vi "Bronkhorst ProPar.vi"() -> ()   [LabVIEW 2015]
doc: "Example VI that demonstrates library features."
uses:
  PL Bronkhorst ProPar.lvclass
panel:
  out "fluid name":string
  out "device model":string
  in  "wink":bool
  in  "reset":bool
  out "temperature, °C":sgl
  out "sensor type":u8(ring) items=["pressure (controller)"=0, "liquid volume (controller)"=1, "liquid/gas mass (controller)"=2, "gas volume (controller)"=3, "other sensor type (controller)"=4, "pressure (sensor)"=128, "liquid volume (sensor)"=129, "liquid/gas mass (sensor)"=130, "gas volume (sensor)"=131, "other sensor type (sensor)"=132]
  out "device type":string
  in  "control mode":u8(ring) items=["setpoint = BUS setpoint", "setpoint = analog input", "setpoint = master output(FLOW-BUS) * slave factor(FLOW-BUS)", "close valve", "controller idle", "testmode enable", "tuningmode enable", "setpoint = 100%", "purge valve", "calibration mode enable", "setpoint = master output(analog in) * slave factor(FLOW-BUS)", "setpoint = keyboard OR FLOW-BUS setpoint", "setpoint = 0%", "setpoint = master output(FLOW-BUS) * slave factor(analog in)", "(FPP) range select mode", "(FPP) manual start sensor select, automatic end sensor", "(FPP) automatic start sensor select, manual end sensor", "(FPP) automatic start and end sensor", "setpoint = RS232 setpoint", "RS232 broadcast mode", "valve stearing", "analog valve stearing", "valve safe state"]
  out "counter unit":string
  in  "counter value":sgl
  out "capacity":sgl
  in  "setpoint":sgl
  out "capacity unit":string
  out "measured value":sgl
  out "firmware version":string
  in  "user tag":string
  out "id string":string
  in  "node":u8
  out "ProPar":refnum<class "PL Bronkhorst ProPar.lvclass">
  in  "baud rate":u32=38400
  in  "port":refnum<visa-resource-name>
  out "error":errorcluster
  in  "stop":bool
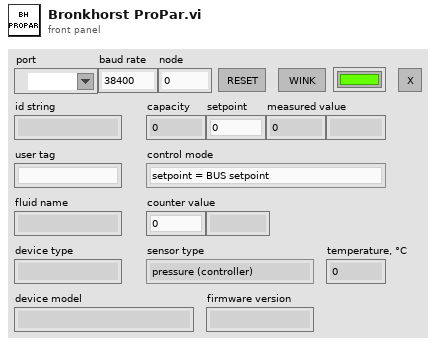
[diagram p1: front panel]
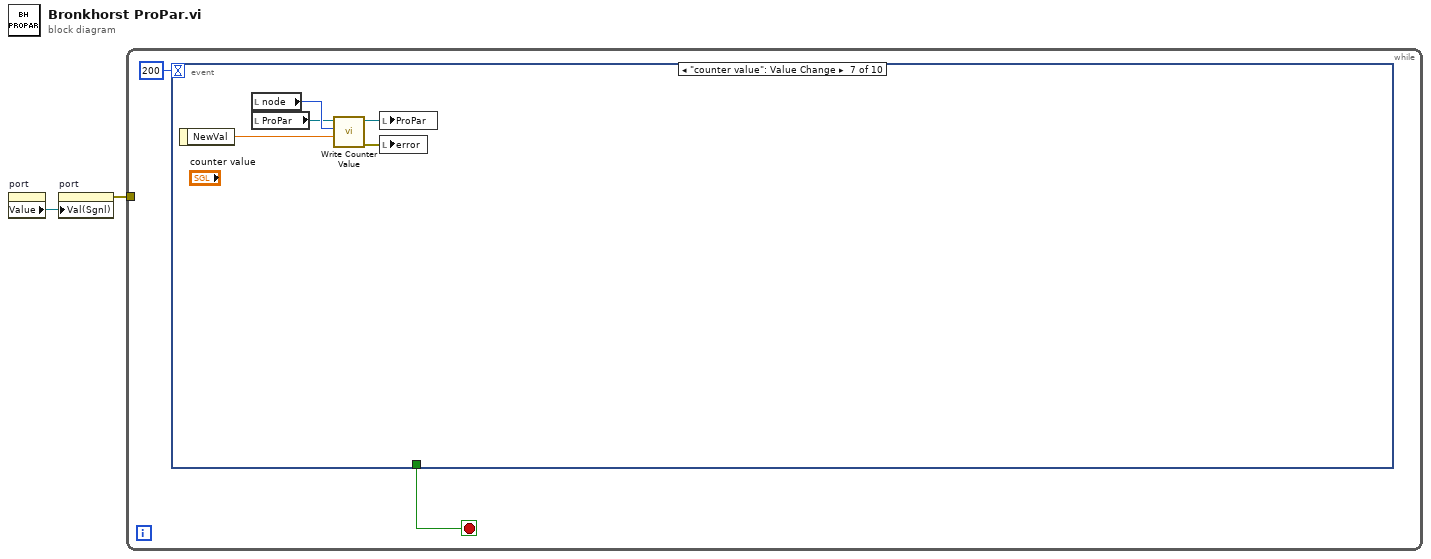
[diagram p0: block diagram]
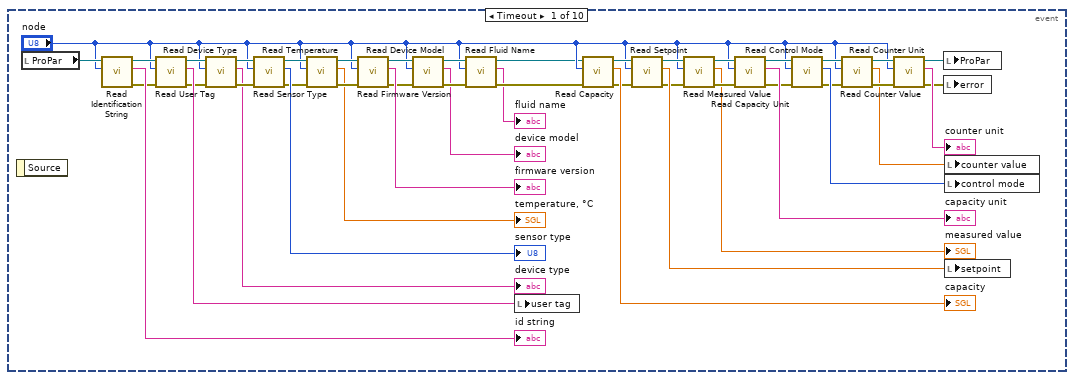
[diagram p2: hidden frame]
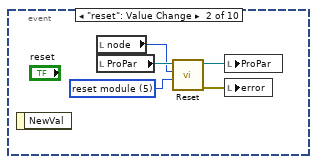
[diagram p3: hidden frame]
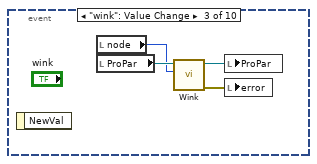
[diagram p4: hidden frame]
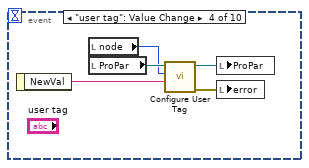
[diagram p5: hidden frame]
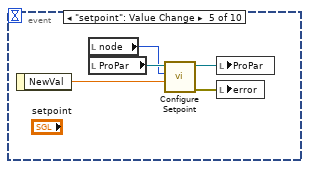
[diagram p6: hidden frame]
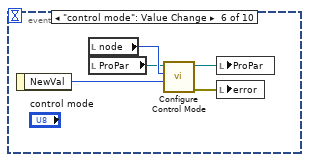
[diagram p7: hidden frame]
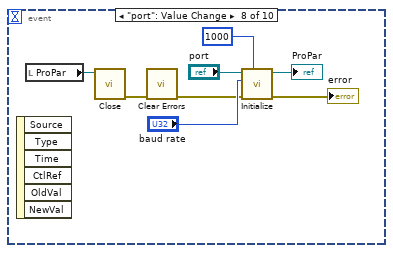
[diagram p8: hidden frame]
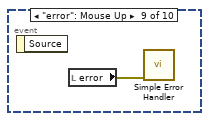
[diagram p9: hidden frame]
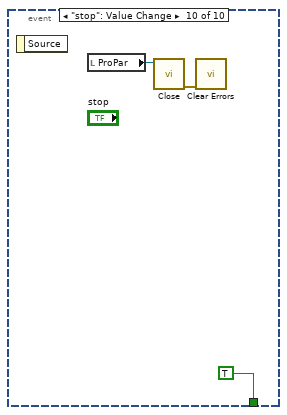
[diagram p10: hidden frame]
diagram:
  n1 = property on="port" class="VISAName"() -> ("Value"=w1:refnum<visa-resource-name>)  [unwired: 2 in, 2 out]
  n2 = property on="port" class="VISAName"("Val(Sgnl)"=w1) -> (error out=w2:errorcluster)  [unwired: 2 in, 1 out]
  n3 = while {
    tunnel: w2 -> [_]
    stop <- w3 stop-if-true
    n4 = event shown="[6] \"counter value\": Value Change" {
      selector: _ -> [_ _ _ _ _ _ _ _ _ _]
      dyn-events: _ -> [_ _ _ _ _ _ _ _ _ _]
      timeout: 200 -> [_ _ _ _ _ _ _ _ _ _]
      tunnel: [_ _ _ _ _ _ _ _ _ TRUE ("stop")] -> w3
      event Timeout {
        n5 = event-data() -> ()  [unwired: 1 in, 1 out]
        n6 = local read "ProPar"() -> (w51:refnum<class "PL Bronkhorst ProPar.lvclass">)
        n7 = call "Read Identification String.vi"("node"="node", "ProPar in"=w51) -> ("error out"=w46:errorcluster, "id string"=→"id string":string, "ProPar out"=w49:refnum<class "PL Bronkhorst ProPar.lvclass">)  [unwired: 7 in]
        n8 = call "Read User Tag.vi"("error in (no error)"=w46, "node"="node", "ProPar in"=w49) -> ("error out"=w44:errorcluster, "user tag"=w48:string, "ProPar out"=w45:refnum<class "PL Bronkhorst ProPar.lvclass">)  [unwired: 6 in]
        n9 = call "Read Device Type.vi"("error in (no error)"=w44, "node"="node", "ProPar in"=w45) -> ("error out"=w42:errorcluster, "device type"=→"device type":string, "ProPar out"=w43:refnum<class "PL Bronkhorst ProPar.lvclass">)  [unwired: 6 in]
        n10 = call "Read Sensor Type.vi"("error in (no error)"=w42, "node"="node", "ProPar in"=w43) -> ("error out"=w38:errorcluster, "sensor type"=→"sensor type":u8, "ProPar out"=w39:refnum<class "PL Bronkhorst ProPar.lvclass">)  [unwired: 6 in]
        n11 = call "Read Temperature.vi"("error in (no error)"=w38, "node"="node", "ProPar in"=w39) -> ("error out"=w36:errorcluster, "temperature, °C"=→"temperature, °C":sgl, "ProPar out"=w37:refnum<class "PL Bronkhorst ProPar.lvclass">)  [unwired: 6 in]
        n12 = call "Read Firmware Version.vi"("error in (no error)"=w36, "node"="node", "ProPar in"=w37) -> ("error out"=w13:errorcluster, "firmware version"=→"firmware version":string, "ProPar out"=w14:refnum<class "PL Bronkhorst ProPar.lvclass">)  [unwired: 6 in]
        n13 = call "Read Device Model.vi"("error in (no error)"=w13, "node"="node", "ProPar in"=w14) -> ("error out"=w10:errorcluster, "device model"=→"device model":string, "ProPar out"=w12:refnum<class "PL Bronkhorst ProPar.lvclass">)  [unwired: 6 in]
        n14 = call "Read Fluid Name.vi"("error in (no error)"=w10, "node"="node", "ProPar in"=w12) -> ("error out"=w9:errorcluster, "fluid name"=→"fluid name":string, "ProPar out"=w8:refnum<class "PL Bronkhorst ProPar.lvclass">)  [unwired: 6 in]
        n15 = local write "user tag"(w48) -> ()
        n16 = call "Read Capacity.vi"("error in (no error)"=w9, "node"="node", "ProPar in"=w8) -> ("error out"=w26:errorcluster, "capacity"=→"capacity":sgl, "ProPar out"=w30:refnum<class "PL Bronkhorst ProPar.lvclass">)  [unwired: 6 in]
        n17 = call "Read Setpoint.vi"("error in (no error)"=w26, "node"="node", "ProPar in"=w30) -> ("error out"=w27:errorcluster, "setpoint"=w28:sgl, "ProPar out"=w25:refnum<class "PL Bronkhorst ProPar.lvclass">)  [unwired: 6 in]
        n18 = call "Read Measured Value.vi"("error in (no error)"=w27, "node"="node", "ProPar in"=w25) -> ("error out"=w33:errorcluster, "measured value"=→"measured value":sgl, "ProPar out"=w34:refnum<class "PL Bronkhorst ProPar.lvclass">)  [unwired: 6 in]
        n19 = call "Read Capacity Unit.vi"("error in (no error)"=w33, "node"="node", "ProPar in"=w34) -> ("error out"=w23:errorcluster, "capacity unit"=→"capacity unit":string, "ProPar out"=w24:refnum<class "PL Bronkhorst ProPar.lvclass">)  [unwired: 6 in]
        n20 = call "Read Control Mode.vi"("error in (no error)"=w23, "node"="node", "ProPar in"=w24) -> ("error out"=w15:errorcluster, "control mode"=w22:u8, "ProPar out"=w20:refnum<class "PL Bronkhorst ProPar.lvclass">)  [unwired: 6 in]
        n21 = call "Read Counter Value.vi"("error in (no error)"=w15, "node"="node", "ProPar in"=w20) -> ("error out"=w16:errorcluster, "counter value"=w5:sgl, "ProPar out"=w19:refnum<class "PL Bronkhorst ProPar.lvclass">)  [unwired: 6 in]
        n22 = call "Read Counter Unit.vi"("error in (no error)"=w16, "node"="node", "ProPar in"=w19) -> ("error out"=w17:errorcluster, "counter unit"=→"counter unit":string, "ProPar out"=w18:refnum<class "PL Bronkhorst ProPar.lvclass">)  [unwired: 6 in]
        n23 = local write "ProPar"(w18) -> ()
        n24 = local write "error"(w17) -> ()
        n25 = local write "counter value"(w5) -> ()
        n26 = local write "control mode"(w22) -> ()
        n27 = local write "setpoint"(w28) -> ()
      }
      event "reset": Value Change {
        w52 = u8 5 items=["reset counter value"=1, "reset alarm"=2, "restart batch counter"=3, "reset counter value (counter off)"=4, "reset module"=5] ("command")
        n28 = event-data() -> ()  [unwired: 1 in, 1 out]
        n29 = local read "node"() -> (w53:u8)
        n30 = local read "ProPar"() -> (w54:refnum<class "PL Bronkhorst ProPar.lvclass">)
        n31 = call "Reset.vi"("command"=w52, "node"=w53, "ProPar in"=w54) -> ("error out"=w55:errorcluster, "ProPar out"=w56:refnum<class "PL Bronkhorst ProPar.lvclass">)  [unwired: 7 in]
        n32 = local write "ProPar"(w56) -> ()
        n33 = local write "error"(w55) -> ()
      }
      event "wink": Value Change {
        n34 = event-data() -> ()  [unwired: 1 in, 1 out]
        n35 = local read "node"() -> (w57:u8)
        n36 = local read "ProPar"() -> (w58:refnum<class "PL Bronkhorst ProPar.lvclass">)
        n37 = call "Wink.vi"("node"=w57, "ProPar in"=w58) -> ("error out"=w59:errorcluster, "ProPar out"=w60:refnum<class "PL Bronkhorst ProPar.lvclass">)  [unwired: 8 in]
        n38 = local write "ProPar"(w60) -> ()
        n39 = local write "error"(w59) -> ()
      }
      event "user tag": Value Change {
        n40 = event-data() -> ("NewVal"=w61:string)  [unwired: 1 in]
        n41 = local read "node"() -> (w62:u8)
        n42 = local read "ProPar"() -> (w65:refnum<class "PL Bronkhorst ProPar.lvclass">)
        n43 = call "Configure User Tag.vi"("user tag"=w61, "node"=w62, "ProPar in"=w65) -> ("error out"=w63:errorcluster, "ProPar out"=w64:refnum<class "PL Bronkhorst ProPar.lvclass">)  [unwired: 7 in]
        n44 = local write "ProPar"(w64) -> ()
        n45 = local write "error"(w63) -> ()
      }
      event "setpoint": Value Change {
        n46 = event-data() -> ("NewVal"=w68:sgl)  [unwired: 1 in]
        n47 = local read "node"() -> (w66:u8)
        n48 = local read "ProPar"() -> (w67:refnum<class "PL Bronkhorst ProPar.lvclass">)
        n49 = call "Configure Setpoint.vi"("setpoint"=w68, "node"=w66, "ProPar in"=w67) -> ("error out"=w69:errorcluster, "ProPar out"=w70:refnum<class "PL Bronkhorst ProPar.lvclass">)  [unwired: 7 in]
        n50 = local write "ProPar"(w70) -> ()
        n51 = local write "error"(w69) -> ()
      }
      event "control mode": Value Change {
        n52 = event-data() -> ("NewVal"=w73:u8)  [unwired: 1 in]
        n53 = local read "node"() -> (w72:u8)
        n54 = local read "ProPar"() -> (w71:refnum<class "PL Bronkhorst ProPar.lvclass">)
        n55 = call "Configure Control Mode.vi"("control mode"=w73, "node"=w72, "ProPar in"=w71) -> ("error out"=w74:errorcluster, "ProPar out"=w75:refnum<class "PL Bronkhorst ProPar.lvclass">)  [unwired: 7 in]
        n56 = local write "ProPar"(w75) -> ()
        n57 = local write "error"(w74) -> ()
      }
      event "counter value": Value Change {
        n58 = event-data() -> ("NewVal"=w76:sgl)  [unwired: 1 in]
        n59 = local read "node"() -> (w78:u8)
        n60 = local read "ProPar"() -> (w77:refnum<class "PL Bronkhorst ProPar.lvclass">)
        n61 = call "Write Counter Value.vi"("counter value"=w76, "node"=w78, "ProPar in"=w77) -> ("error out"=w79:errorcluster, "ProPar out"=w80:refnum<class "PL Bronkhorst ProPar.lvclass">)  [unwired: 7 in]
        n62 = local write "ProPar"(w80) -> ()
        n63 = local write "error"(w79) -> ()
      }
      event "port": Value Change {
        n64 = event-data() -> ()  [unwired: 1 in, 6 out]
        n65 = local read "ProPar"() -> (w83:refnum<class "PL Bronkhorst ProPar.lvclass">)
        n66 = call "Close.vi"("ProPar in"=w83) -> ("error out"=w85:errorcluster)  [unwired: 10 in]
        n67 = call <vilib>:"Clear Errors.vi"("error in (no error)"=w85) -> ("error out"=w82:errorcluster)  [unwired: 5 in, 1 out]
        n68 = call "Initialize.vi"("timeout, ms (1000)"=u32 1000, "error in (no error)"=w82, "baud rate (38400)"="baud rate", "port"="port") -> ("error out"=→"error":errorcluster, "ProPar out"=→"ProPar":refnum<class "PL Bronkhorst ProPar.lvclass">)  [unwired: 6 in]
      }
      event "error": Mouse Up {
        n69 = event-data() -> ()  [unwired: 1 in, 1 out]
        n70 = local read "error"() -> (w89:errorcluster)
        n71 = call <vilib>:"Simple Error Handler.vi"("error in (no error)"=w89) -> ()  [unwired: 4 in, 5 out]
      }
      event "stop": Value Change {
        n72 = event-data() -> ()  [unwired: 1 in, 1 out]
        n73 = local read "ProPar"() -> (w91:refnum<class "PL Bronkhorst ProPar.lvclass">)
        n74 = call "Close.vi"("ProPar in"=w91) -> ("error out"=w90:errorcluster)  [unwired: 10 in]
        n75 = call <vilib>:"Clear Errors.vi"("error in (no error)"=w90) -> ()  [unwired: 5 in, 2 out]
      }
    }
  }
